vi "Calc_Btm.vi"(8 "Draw?":bool, 10 "Edge Points":cluster{dbl, dbl}[][](array[cluster]), 11 "picture in":picture) -> (2 "Bottom grid":cluster{"x":dbl, "y":dbl}[][](array[cluster]), 3 "picture out":picture)   [LabVIEW 2022 SP3]
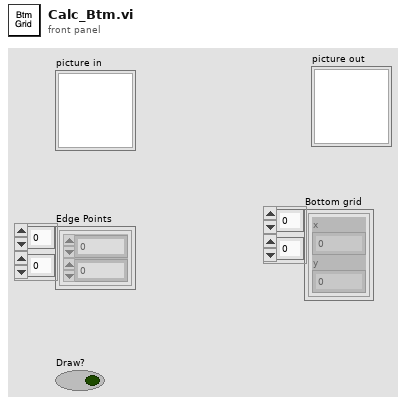
[diagram p1: front panel]
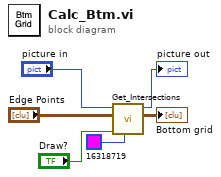
[diagram p0: block diagram]
diagram:
  n1 = call "Get_Intersections.vi"("color"=u32 16318719, "Draw?"="Draw?", "Edge Points"="Edge Points", "picture in"="picture in") -> ("All Points"=→"Bottom grid":cluster{"x":dbl, "y":dbl}[][], "picture out"=→"picture out":picture)  [unwired: 6 in]
